vi "Coercion.vi"(7 "Robot Width (in)":dbl, 8 "Backarm Length (in)":dbl, 9 "Forearm Length (in)":dbl, 10 "Beta":dbl, 11 "Alpha":dbl) -> (2 "New Beta":dbl, 3 "New Alpha":dbl)   [LabVIEW 2017]
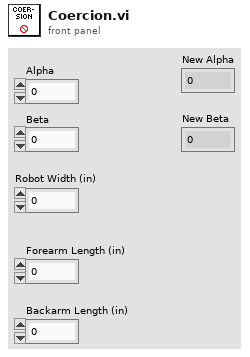
[diagram p1: front panel]
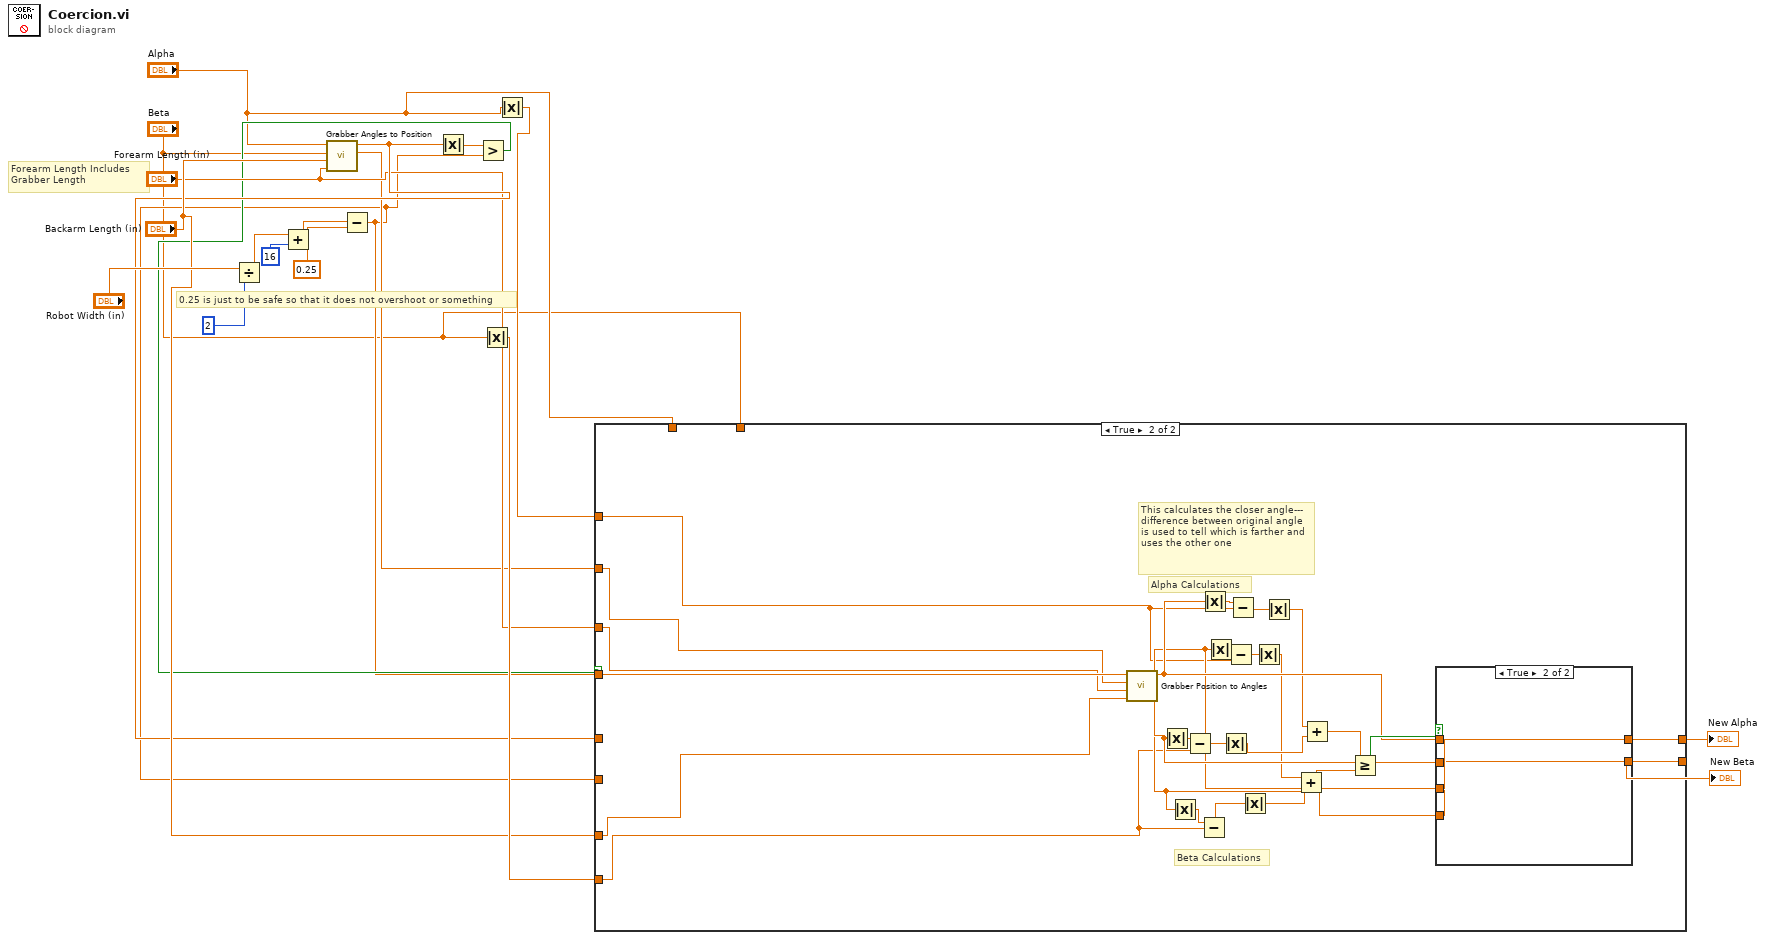
[diagram p0: block diagram]
diagram:
  # "0.25 is just to be safe so that it does not overshoot or something"
  # "Forearm Length Includes Grabber Length"
  n1 = Divide(x="Robot Width (in)", y=2) -> (x/y=w17:dbl)
  n2 = Add(x=w17, y=16) -> (x+y=w15:dbl)
  n3 = call "Grabber Angles to Position.vi"("Forerm Length"="Forearm Length (in)", "Backarm Length"="Backarm Length (in)", "Forearm Angle Degrees"="Beta", "Backarm Angle Degrees"="Alpha") -> ("Y Final"=w7:dbl, "X Final"=w10:dbl)  [unwired: 6 in]
  n4 = Subtract(x=w15, y=0.25) -> (x-y=w5:dbl)
  n5 = Absolute Value(x=w10) -> (abs(x)=w13:dbl)
  n6 = Greater?(x=w13, y=w5) -> (0:w8:bool)
  n7 = Absolute Value(x="Beta") -> (abs(x)=w12:dbl)
  n8 = Absolute Value(x="Alpha") -> (abs(x)=w6:dbl)
  n9 = case shown="True" w8 {
    tunnel: w12 -> [_ w29]
    tunnel: "Backarm Length (in)" -> [_ w28]
    tunnel: w5 -> [_ _]
    tunnel: w10 -> [_ _]
    tunnel: "Forearm Length (in)" -> [_ w26]
    tunnel: w7 -> [_ w25]
    tunnel: w6 -> [_ w24]
    tunnel: w5 -> [_ w27]
    tunnel: [w21 w23] -> w4
    tunnel: [w20 w22] -> w3
    tunnel: "Alpha" -> [w21 _]
    tunnel: "Beta" -> [w20 _]
    frame False {
    }
    frame True {
      # "Beta Calculations"
      # "Alpha Calculations"
      # "This calculates the closer angle--- difference between original angle is used to tell which is farther and uses the other one"
      n10 = call "Grabber Position to Angles.vi"("Backarm Length"=w28, "Forearm Length"=w26, "Y Initial"=w25, "X Initial"=w27) -> ("Forearm Angle\nDegrees 2"=w38:dbl, "Backarm Angle\nDegrees 2"=w43:dbl, "Forearm Angle\nDegrees 1"=w44:dbl, "Backarm Angle\nDegrees 1"=w45:dbl)  [unwired: 4 in]
      n11 = Absolute Value(x=w44) -> (abs(x)=w36:dbl)
      n12 = Absolute Value(x=w38) -> (abs(x)=w37:dbl)
      n13 = Subtract(x=w36, y=w29) -> (x-y=w39:dbl)
      n14 = Subtract(x=w37, y=w29) -> (x-y=w40:dbl)
      n15 = Absolute Value(x=w45) -> (abs(x)=w34:dbl)
      n16 = Absolute Value(x=w43) -> (abs(x)=w35:dbl)
      n17 = Absolute Value(x=w39) -> (abs(x)=w33:dbl)
      n18 = Subtract(x=w35, y=w24) -> (x-y=w41:dbl)
      n19 = Subtract(x=w34, y=w24) -> (x-y=w42:dbl)
      n20 = Absolute Value(x=w40) -> (abs(x)=w30:dbl)
      n21 = Absolute Value(x=w41) -> (abs(x)=w32:dbl)
      n22 = Absolute Value(x=w42) -> (abs(x)=w31:dbl)
      n23 = Add(x=w32, y=w30) -> (x+y=w46:dbl)
      n24 = Add(x=w31, y=w33) -> (x+y=w47:dbl)
      n25 = Greater Or Equal?(x=w47, y=w46) -> (x >= y?=w48:bool)
      n26 = case shown="True" w48 {
        tunnel: w45 -> [w50 _]
        tunnel: w44 -> [w49 _]
        tunnel: w43 -> [_ w52]
        tunnel: w38 -> [_ w51]
        tunnel: [w50 w52] -> w23
        tunnel: [w49 w51] -> w22
        frame False {
        }
        frame True {
        }
      }
    }
  }
  "New Alpha" <- w4
  "New Beta" <- w3
